vi "Configure Units.vi"(0 "VISA resource name":refnum<visa-resource-name>, 1 "Enable User Defined Pressure":bool, 5 "Flow Units (0: Sccm)":u16(ring) items=["Sccm", "Slm", "Slh", "Scfm", "Scfh", "Sm3m", "Sm3h"], 7 "Temperature Units (0: Celsius)":u16(ring) items=["Celsius", "Fahrenheit"], 9 "Pressure Units (1: Kilo Pascals)":u16(ring)=1 items=["Pascals", "Kilo Pascals", "Mili Pascals", "Mili Bar", "Bar", "mmHg", "mmWa", "Psi", "Psf", "inHg", "inWg", "Kcm2"], 11 "error in (no error)":errorcluster, 12 "Pressure Unit Identifier":string, 13 "Pressure Unit Coefficient":dbl) -> (4 "VISA resource name out":refnum<visa-resource-name>, 15 "error out":errorcluster)   [LabVIEW 2023, in "Fluke Molbox 1 Plus.lvlib"]
doc: "Configure different kinds of units."
uses:
  Fluke Molbox 1 Plus.lvlib
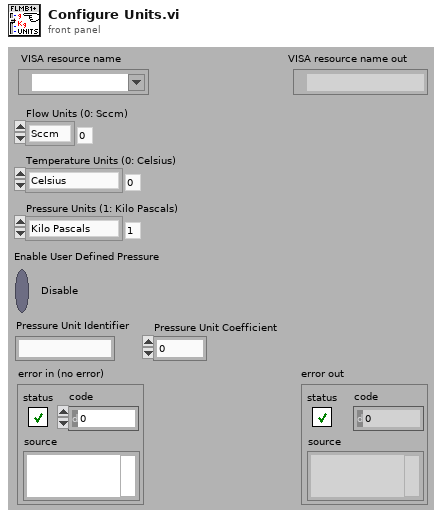
[diagram p1: front panel]
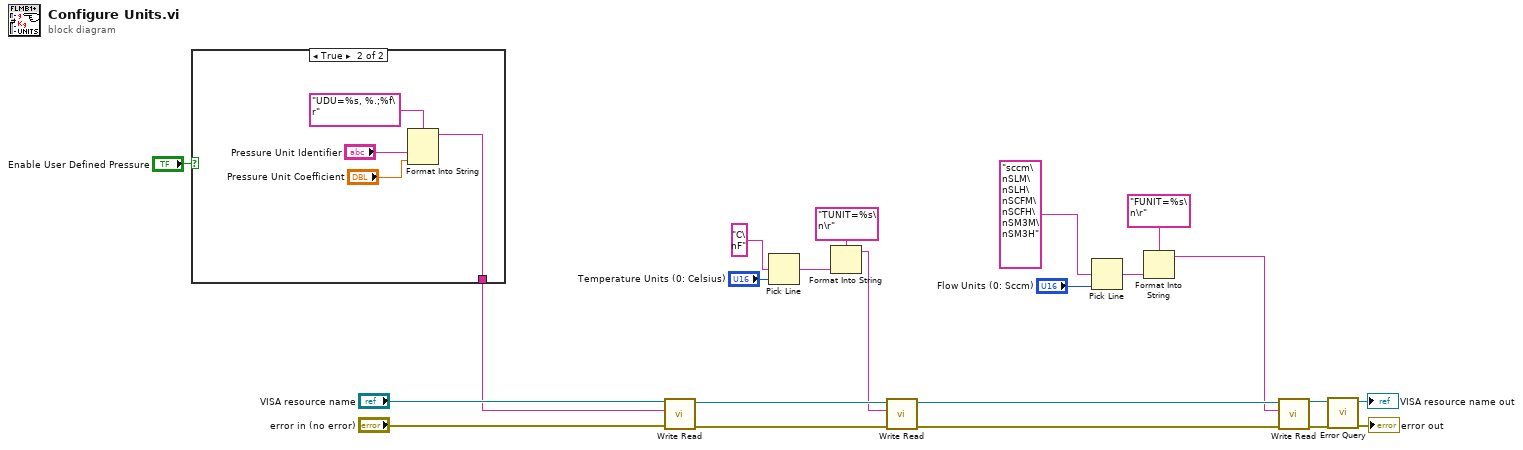
[diagram p0: block diagram]
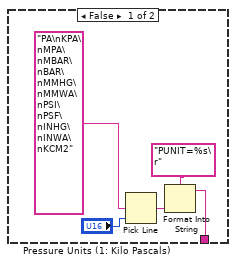
[diagram p2: hidden frame]
diagram:
  n1 = case shown="True" "Enable User Defined Pressure" {
    tunnel: [w25 w28] -> w10
    frame False {
      n2 = Pick Line(multi-line string="PA\nKPA\nMPA\nMBAR\nBAR\nMMHG\nMMWA\nPSI\nPSF\nINHG\nINWA\nKCM2", line index="Pressure Units (1: Kilo Pascals)") -> (output string=w27:string)  [unwired: 1 in]
      n3 = Format Into String(format string="PUNIT=%s\r", w27) -> (resulting string=w25:string)  [unwired: 2 in, 1 out]
    }
    frame True {
      n4 = Format Into String(format string="UDU=%s, %.;%f\r", "Pressure Unit Identifier", "Pressure Unit Coefficient") -> (resulting string=w28:string)  [unwired: 2 in, 1 out]
    }
  }
  n5 = call "Write Read.vi"("error in (no error)"="error in (no error)", "Write String"=w10, "VISA resource name"="VISA resource name") -> ("error out"=w8:errorcluster, "VISA resource name out"=w7:refnum<visa-resource-name>)  [unwired: 6 in, 1 out]
  n6 = Pick Line(multi-line string="C\nF", line index="Temperature Units (0: Celsius)") -> (output string=w21:string)  [unwired: 1 in]
  n7 = Format Into String(format string="TUNIT=%s\n\r", w21) -> (resulting string=w6:string)  [unwired: 2 in, 1 out]
  n8 = call "Write Read.vi"("error in (no error)"=w8, "Write String"=w6, "VISA resource name"=w7) -> ("error out"=w3:errorcluster, "VISA resource name out"=w5:refnum<visa-resource-name>)  [unwired: 6 in, 1 out]
  n9 = Pick Line(multi-line string="sccm\nSLM\nSLH\nSCFM\nSCFH\nSM3M\nSM3H", line index="Flow Units (0: Sccm)") -> (output string=w15:string)  [unwired: 1 in]
  n10 = Format Into String(format string="FUNIT=%s\n\r", w15) -> (resulting string=w4:string)  [unwired: 2 in, 1 out]
  n11 = call "Write Read.vi"("error in (no error)"=w3, "Write String"=w4, "VISA resource name"=w5) -> ("error out"=w1:errorcluster, "VISA resource name out"=w2:refnum<visa-resource-name>)  [unwired: 6 in, 1 out]
  n12 = call "Error Query.vi"("error in (no error)"=w1, "VISA resource name"=w2) -> ("error out"=→"error out":errorcluster, "VISA resource name out"=→"VISA resource name out":refnum<visa-resource-name>)  [unwired: 6 in, 2 out]
